vi "GUI - SET - Triggered Event.vi"(8 "error in (no error)":errorcluster, 10 "Events":T1, 11 "Child_1_Class in":refnum<class "GUI_Class.lvclass">) -> (0 "error out":errorcluster, 3 "Child_1_Class out":refnum<class "GUI_Class.lvclass">)   [LabVIEW 2023, in "GUI_Actor.lvlib" / "GUI_Class.lvclass"]
uses:
  GUI_Class.lvclass
  Usr Ev/GUI - Ctrl - Enum - Events.ctl
  GUI_Class.lvclass/GUI_Class.ctl
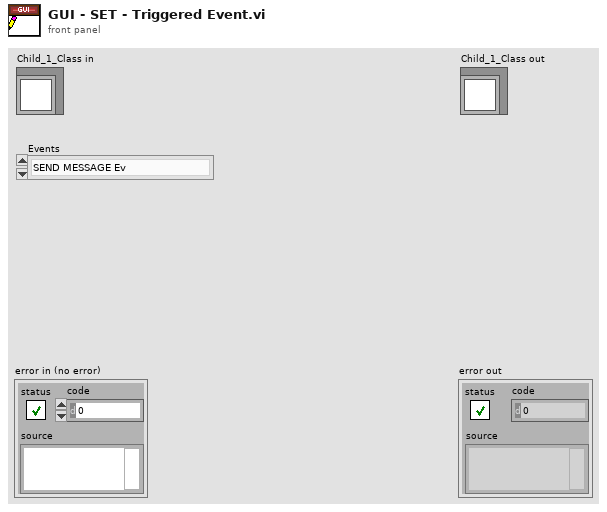
[diagram p1: front panel]
types:
  T1 = typedef "GUI_Actor.lvlib/GUI_Class.lvclass/GUI - Ctrl - Enum - Events.ctl" = enum16{"SEND MESSAGE Ev", "STOP_ACTOR Ev", "INIT_ACTOR Ev", "START Ev", "STOP Ev", "GET Ev", "SET Ev", "ERROR_HANDLER Ev", "RESET Ev", "T2 Ev", "T3 Ev", "T4 Ev"}
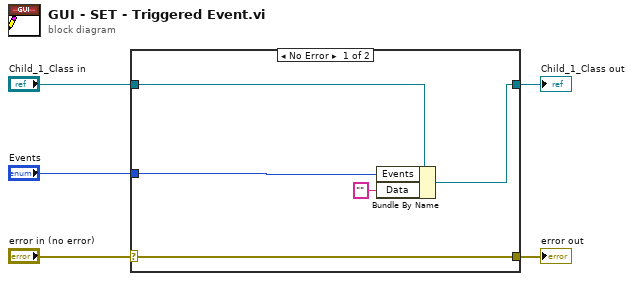
[diagram p0: block diagram]
diagram:
  n1 = case shown="No Error" "error in (no error)" {
    selector: "error in (no error)" -> [w10 w11]
    tunnel: [w10 w11] -> w4
    tunnel: [w8 w12] -> w2
    tunnel: "Child_1_Class in" -> [w9 w12]
    tunnel: "Events" -> [w7 _]
    frame No Error {
      n2 = Bundle By Name(cluster=w9, "Events"=w7, "Data"="" ("Child Trigger Event Cluster.Data")) -> (w8:refnum<class "GUI_Class.lvclass">)
    }
    frame Error {
    }
  }
  "error out" <- w4
  "Child_1_Class out" <- w2
